vi "Desontter _RS232 Com.vi"() -> ()   [LabVIEW 2015]
uses:
  <vilib>/Instr/_visa.llb/VISA Configure Serial Port (Instr).vi
  Galobal variable_TI.vi
panel:
  out "Desontter data 2":i32
  in  "Desontter data":i32
  in  "stop":bool
  out "read buffer":string="\r   0.1        0.0       0.000     07/07/20 10:33:46   Reject"
  out "error out 2":errorcluster
  out "error out":errorcluster
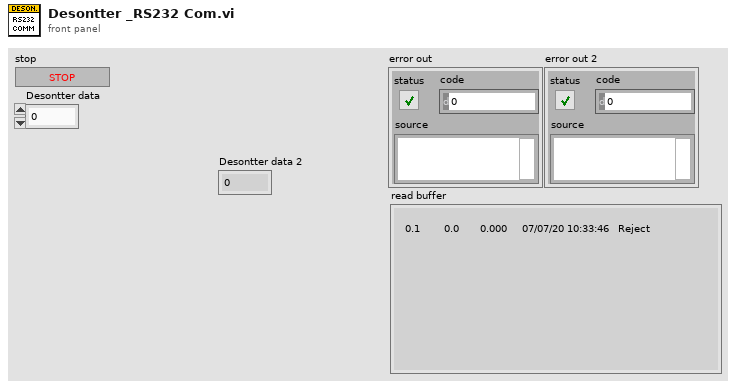
[diagram p1: front panel]
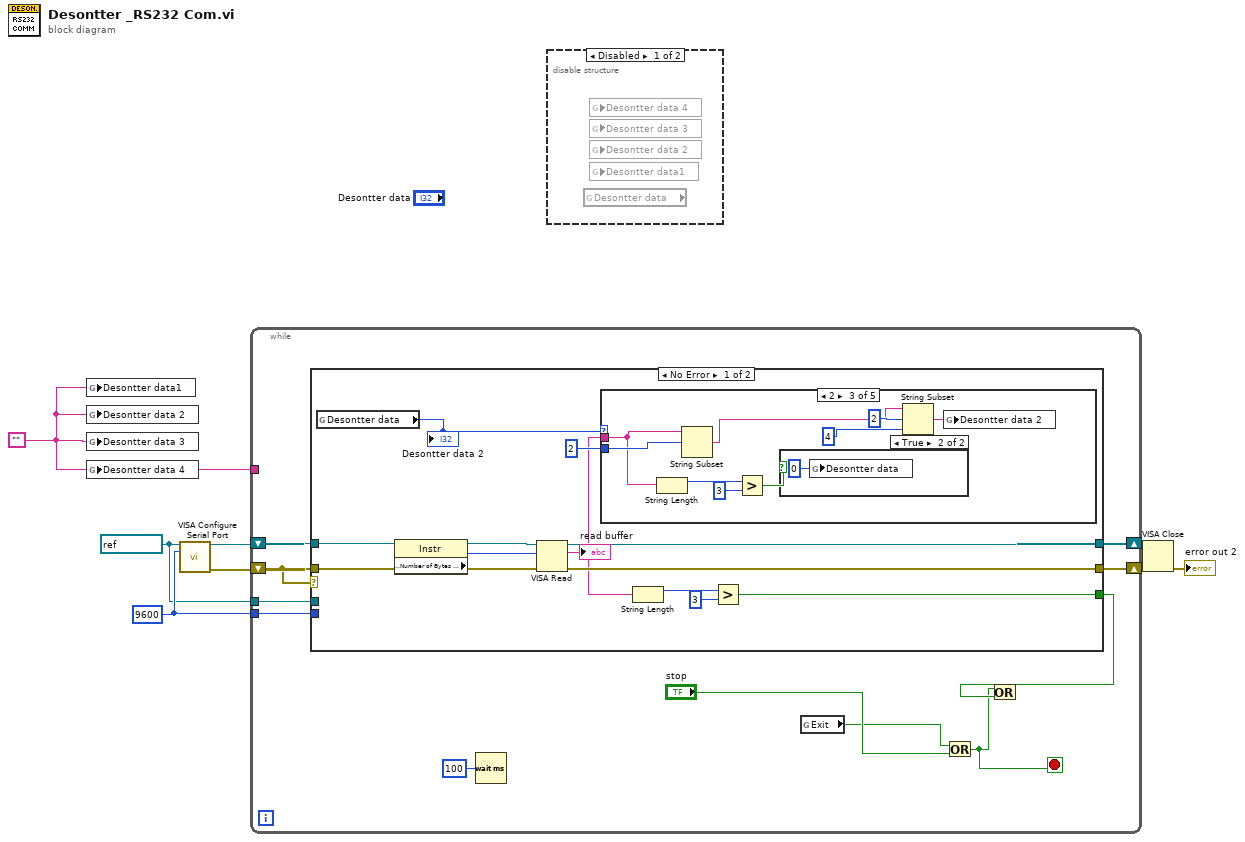
[diagram p0: block diagram]
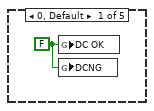
[diagram p3: hidden frame]
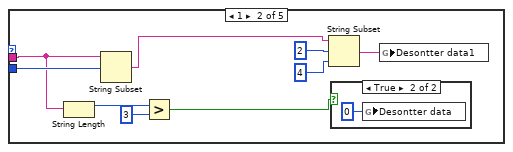
[diagram p4: hidden frame]
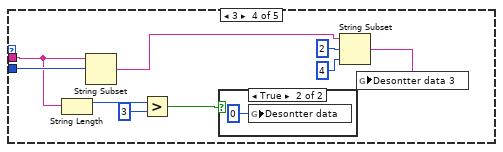
[diagram p7: hidden frame]
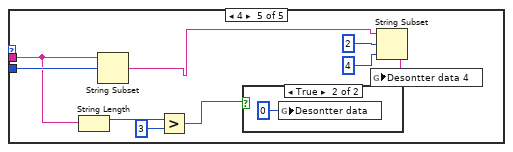
[diagram p9: hidden frame]
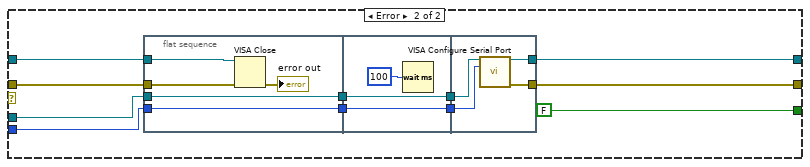
[diagram p11: hidden frame]
diagram:
  w1 = ""
  w3 = u32 9600 ("baud rate (9600)")
  w2 = refnum<visa-resource-name> "COM1" ("VISA resource name")
  n1 = global write "Galobal variable_TI.vi" "Desontter data1"(w1) -> ()
  n2 = global write "Galobal variable_TI.vi" "Desontter data 2"(w1) -> ()
  n3 = global write "Galobal variable_TI.vi" "Desontter data 3"(w1) -> ()
  n4 = global write "Galobal variable_TI.vi" "Desontter data 4"(w1) -> ()
  n5 = call-poly "VISA Configure Serial Port"("VISA resource name"=w2, "baud rate (9600)"=w3) -> ("VISA resource name out"=w8:refnum<visa-resource-name>, "error out"=w7:errorcluster)  [unwired: 12 in]
  n6 = while {
    shift-right: [w17] -> w5
    shift-left: w8 -> [w19]
    shift-right: [w16] -> w4
    shift-left: w7 -> [w18]
    tunnel: w3 -> [w15]
    tunnel: w2 -> [w14]
    tunnel: w1 -> [_]
    stop <- w9 stop-if-true
    n7 = case shown="No Error" w18 {
      tunnel: w19 -> [w29 w83]
      tunnel: w18 -> [w28 w84]
      tunnel: [w27 w82] -> w17
      tunnel: [w26 w81] -> w16
      tunnel: w15 -> [_ w78]
      tunnel: w14 -> [_ w75]
      tunnel: [w23 FALSE] -> w10
      frame No Error {
        n8 = global read "Galobal variable_TI.vi" "Desontter data"() -> (w22:i32)
        "Desontter data 2" <- w22
        n9 = property class="Instr"(reference=w29, error in=w28) -> (reference out=w32:refnum<visa-resource-name>, error out=w31:errorcluster, "Serial Settings:Number of Bytes at Serial Port"=w30:u32)
        n10 = VISA Read(VISA resource name=w32, byte count=w30, error in (no error)=w31) -> (VISA resource name out=w27:refnum<visa-resource-name>, read buffer=w20:string, error out=w26:errorcluster)  [unwired: 1 out]
        "read buffer" <- w20
        n11 = case shown="2" w22 {
          tunnel: 2 ("length (rest)") -> [_ w42 w52 w62 w72]
          tunnel: w20 -> [_ w35 w46 w55 w65]
          frame 0, Default {
            w33 = FALSE ("DC OK")
            n12 = global write "Galobal variable_TI.vi" "DC OK"(w33) -> ()
            n13 = global write "Galobal variable_TI.vi" "DCNG"(w33) -> ()
          }
          frame 1 {
            n14 = String Length(string=w35) -> (length=w36:i32)
            n15 = String Subset(string=w35, offset (0)=w42) -> (substring=w39:string)  [unwired: 1 in]
            n16 = Greater?(x=w36, y=3) -> (0:w34:bool)
            n17 = String Subset(string=w39, offset (0)=2, length (rest)=4 ("length (rest)")) -> (substring=w38:string)
            n18 = case shown="True" w34 {
              frame False {
              }
              frame True {
                n19 = global write "Galobal variable_TI.vi" "Desontter data"(0 ("Desontter data")) -> ()
              }
            }
            n20 = global write "Galobal variable_TI.vi" "Desontter data1"(w38) -> ()
          }
          frame 2 {
            n21 = String Length(string=w46) -> (length=w47:i32)
            n22 = String Subset(string=w46, offset (0)=w52) -> (substring=w50:string)  [unwired: 1 in]
            n23 = Greater?(x=w47, y=3) -> (0:w45:bool)
            n24 = case shown="True" w45 {
              frame False {
              }
              frame True {
                n25 = global write "Galobal variable_TI.vi" "Desontter data"(0 ("Desontter data")) -> ()
              }
            }
            n26 = String Subset(string=w50, offset (0)=2, length (rest)=4 ("length (rest)")) -> (substring=w49:string)
            n27 = global write "Galobal variable_TI.vi" "Desontter data 2"(w49) -> ()
          }
          frame 3 {
            n28 = String Length(string=w55) -> (length=w56:i32)
            n29 = String Subset(string=w55, offset (0)=w62) -> (substring=w59:string)  [unwired: 1 in]
            n30 = Greater?(x=w56, y=3) -> (0:w54:bool)
            n31 = case shown="True" w54 {
              frame False {
              }
              frame True {
                n32 = global write "Galobal variable_TI.vi" "Desontter data"(0 ("Desontter data")) -> ()
              }
            }
            n33 = String Subset(string=w59, offset (0)=2, length (rest)=4 ("length (rest)")) -> (substring=w58:string)
            n34 = global write "Galobal variable_TI.vi" "Desontter data 3"(w58) -> ()
          }
          frame 4 {
            n35 = String Length(string=w65) -> (length=w66:i32)
            n36 = String Subset(string=w65, offset (0)=w72) -> (substring=w69:string)  [unwired: 1 in]
            n37 = Greater?(x=w66, y=3) -> (0:w64:bool)
            n38 = case shown="True" w64 {
              frame False {
              }
              frame True {
                n39 = global write "Galobal variable_TI.vi" "Desontter data"(0 ("Desontter data")) -> ()
              }
            }
            n40 = String Subset(string=w69, offset (0)=2, length (rest)=4 ("length (rest)")) -> (substring=w68:string)
            n41 = global write "Galobal variable_TI.vi" "Desontter data 4"(w68) -> ()
          }
        }
        n42 = String Length(string=w20) -> (length=w25:i32)
        n43 = Greater?(x=w25, y=3) -> (0:w23:bool)
      }
      frame Error {
        n44 = flat-sequence {
          tunnel: w84 -> [w88]
          tunnel: w83 -> [w87]
          tunnel: [w85] -> w79
          tunnel: w78 -> [w86]
          tunnel: [w86] -> w77
          tunnel: w75 -> [w85]
          tunnel: [w91] -> w80
          tunnel: w79 -> [w91]
          tunnel: w77 -> [w90]
          tunnel: [w90] -> w76
          tunnel: [w96] -> w82
          tunnel: [w95] -> w81
          tunnel: w80 -> [w94]
          tunnel: w76 -> [w93]
          frame #0 {
            n45 = VISA Close(VISA resource name=w87, error in (no error)=w88) -> (error out=→"error out":errorcluster)
          }
          frame #1 {
            n46 = Wait (ms)(milliseconds to wait=u32 100) -> ()  [unwired: 1 out]
          }
          frame #2 {
            n47 = call-poly "VISA Configure Serial Port"("VISA resource name"=w94, "baud rate (9600)"=w93) -> ("VISA resource name out"=w96:refnum<visa-resource-name>, "error out"=w95:errorcluster)  [unwired: 12 in]
          }
        }
      }
    }
    n48 = Wait (ms)(milliseconds to wait=u32 100) -> ()  [unwired: 1 out]
    n49 = global read "Galobal variable_TI.vi" "Exit"() -> (w12:bool)
    n50 = Or(x=w12, y="stop") -> (x .or. y?=w9:bool)
    n51 = Or(x=w9, y=w10) -> ()  [unwired: 1 out]
  }
  n52 = disable-structure shown="Disabled" {
    frame Disabled {
      n53 = global read "Galobal variable_TI.vi" "Desontter data"() -> ()  [unwired: 1 out]
      n54 = global read "Galobal variable_TI.vi" "Desontter data 4"() -> ()  [unwired: 1 in]
      n55 = global read "Galobal variable_TI.vi" "Desontter data 3"() -> ()  [unwired: 1 in]
      n56 = global read "Galobal variable_TI.vi" "Desontter data 2"() -> ()  [unwired: 1 in]
      n57 = global read "Galobal variable_TI.vi" "Desontter data1"() -> ()  [unwired: 1 in]
    }
    frame Enabled {
    }
  }
  n58 = VISA Close(VISA resource name=w5, error in (no error)=w4) -> (error out=→"error out 2":errorcluster)
